vi "pulse detector tester_host vi.vi"() -> ()   [LabVIEW 2021]
uses:
  FPGA/PDW interpoter params.ctl
  FPGA/reciver params.ctl
  <vilib>/FPGAPlugInAG/USRP 294xR; 295xR 200 MSps/niLvFpga_Open_USRP 294xR; 295xR 200 MSps.vi
  <vilib>/rvi/interface/common/dynamic/niFpgaDynamicAddResources.vi
  <vilib>/rvi/interface/common/niFpgaWaitOnOcc.vi
  <vilib>/Utility/error.llb/Error Cluster From Error Code.vi
  <vilib>/rvi/errors/niLvFpgaAdjustHostInterfaceError.vi
  <vilib>/FPGAPlugInAG/Dynamic/niLvFpga_Close_Dynamic.vi
  <vilib>/rvi/interface/nirviOpenFPGA/nirviOpenFPGA.xnode
  FPGA Bitfiles/reciever_USRP294xR;295xR2_pulsedetectormai_nRNCtQH+qRA.lvbitx
  <vilib>/rvi/interface/nirviMethod/nirviMethod.xnode
  <vilib>/rvi/interface/nirviReadWriteControl/nirviReadWriteControl.xnode
  <vilib>/rvi/interface/nirviCloseFPGA/nirviCloseFPGA.xnode
  <vilib>/rvi/errors/niLvFpgaMergeErrorWithErrorCode.vi
  <vilib>/FPGAPlugInAG/Dynamic/niLvFpga_ReadFifo_Dynamic.vi
  NiFpgaLv.dll
  <vilib>/rvi/interface/Simulation/niFpgaSimulationCallBeginRW.vi
  <vilib>/FPGAPlugInAG/Dynamic/niLvFpga_WriteFifo_Dynamic.vi
  <vilib>/FPGAPlugInAG/Dynamic/niLvFpga_ConfigureFifo_Dynamic.vi
panel:
  out "num of pulses detected":i32
  in  "Tab Control 2":T1(tab)
  in  "F base (Hz)":u32 format="%.0p"
  in  "Fs  (Hz)":u32=80000000 format="%.0p"
  in  "Rx max gap (fft cycels)":u8
  in  "Rx max PW (fft cycels)":u16=30000
  in  "Rx min PW (fft cycels)":u16=6
  in  "Rx detection bar (dB)":dbl=120.0
  in  "where the  pulse detector run?":bool caption="run on fpga"
  in  "TDMS IQ file":path=path "C:/Users/NI/Desktop/RDC_chaim.tdms channel0.tdms"
  in  "lo likege removal (bins aruond 0)":i32=-1
  in  "max PW (fft cycels)":dbl=9999.0
  in  "min PW (fft cycels)":u16
  in  "min amp (dB)":dbl format="%_3p"
  out "frequncy resolotion (Hz)":dbl format="%#_3p"
  out "PW_resolotion (sec)":dbl format="%#_6p"
  out "spectrogram":sgl[][](graph)
  in  "Map selector":T2(ring)=enum."inverse grey"
  out "end of file?":bool
  in  "Next Button":bool
  out "PW":cluster{dbl[], dbl[]}(graph)
  out "amp(dB)/ frequncy (Hz)":cluster{dbl[], dbl[]}(graph)
  out "F (Hz)":cluster{dbl[], dbl[]}(graph)
  out "amp(dB)":cluster{dbl[], dbl[]}(graph)
  out "PDWs":T3(array[cluster]) {"t end (sec)" format="%#_6p"; "f(Hz)" format="%#_3p"; "PW (sec)" format="%#_6p"; "magnitude(dB)" format="%#_3g"}
  out "read parts":i32
  in  "off":bool
  out "streaming":bool
  # "Pulse Detector Tester"
  # "resolotions"
  # "This is \"pulse detector\" tester, the user shuold select a TDMS file\nwith some pulses on it and the VI will run it on FPGA or host in \norder to detect the pulses.\nthe reciver params are the parameters needed for the pulse detector:\n max gap - the maxiemom of undetected parts in the spot that \nthe detector keep loking for continuety.\nRx max PW - if the pulse is CW then we like to get  a PDW even if the pulse isnt done.\nRx min PW - less then this size is probbly just termal noise\nRx detection bar - the detection bar.\ndisplay filters could help the user make the presenting graphs easyer to understend."
  # "secnario params"
  # "reciever params"
  # "display filters"
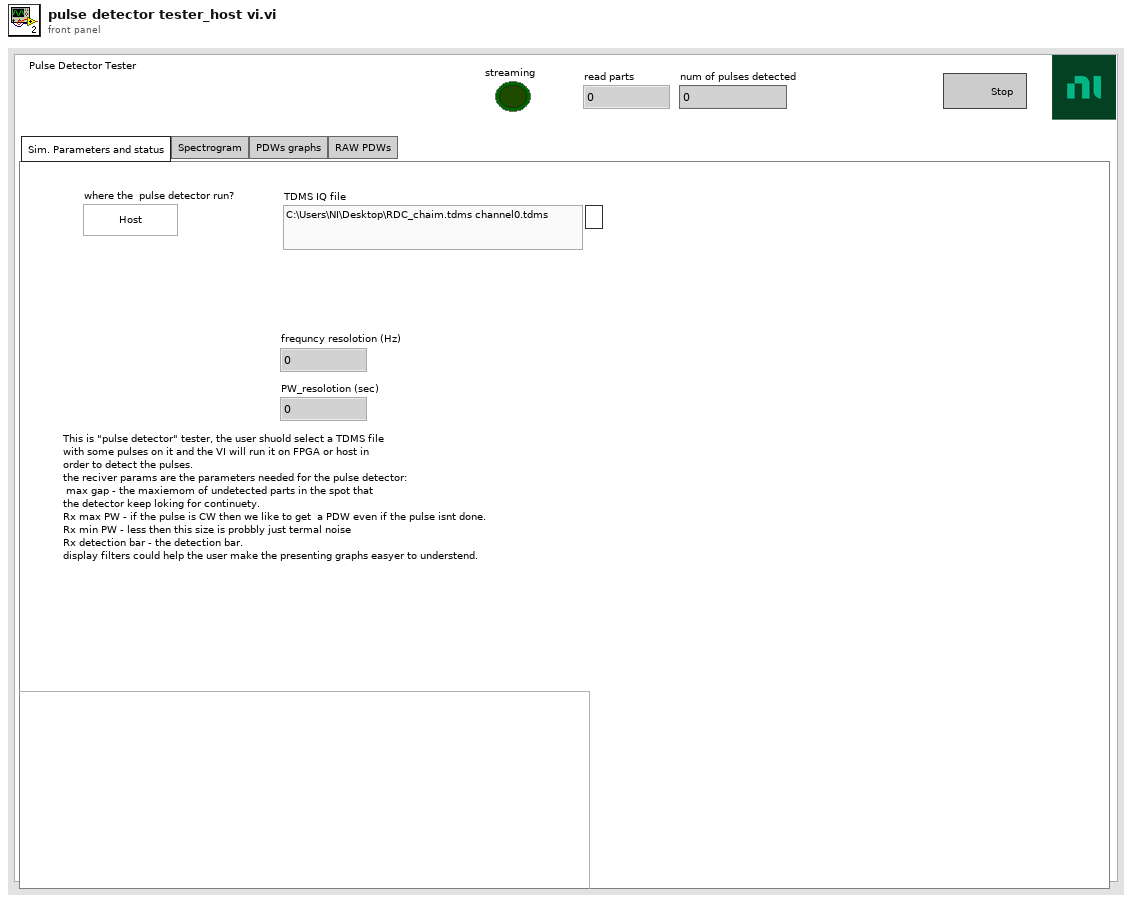
[diagram p1: front panel]
types:
  T1 = enum32{"Sim. Parameters and status", "Spectrogram", "PDWs graphs", "RAW PDWs"}
  T2 = enum16{"fire", "rainbow", "grey", "inverse grey", "ice", "original"}
  T3 = cluster{"f(Hz)":dbl, "PW (sec)":dbl, "magnitude(dB)":dbl, "t end (sec)":dbl}[]
  T4 = enum16{"open", "open or create", "create or replace", "create", "open (read-only)"}
  T5 = typedef "reciver params.ctl" = cluster{"min PW (fft cycels)":u16, "max PW (fft cycels)":u16, "max gap (fft cycels)":u8, "detection bar (liniar amp)":fxp<+,64,63>}
  T6 = typedef "PDW interpoter params.ctl" = cluster{"Fs (Hz)":u32, "fft size ":u32, "F base (Hz)":u32, "min AMP (dB)":dbl, "PW low bar (fft cycle)":dbl, "Pw high bar (fft cycle)":dbl, "lo likege removal (fft bin)":i32, "max gap (fft cycle)":dbl}
  T7 = typedef "specrogram_and_param.ctl" = cluster{"Array out":sgl[][], "start_ time":dbl, "min_amp":dbl, "amp_scale":dbl, "end of file":bool}
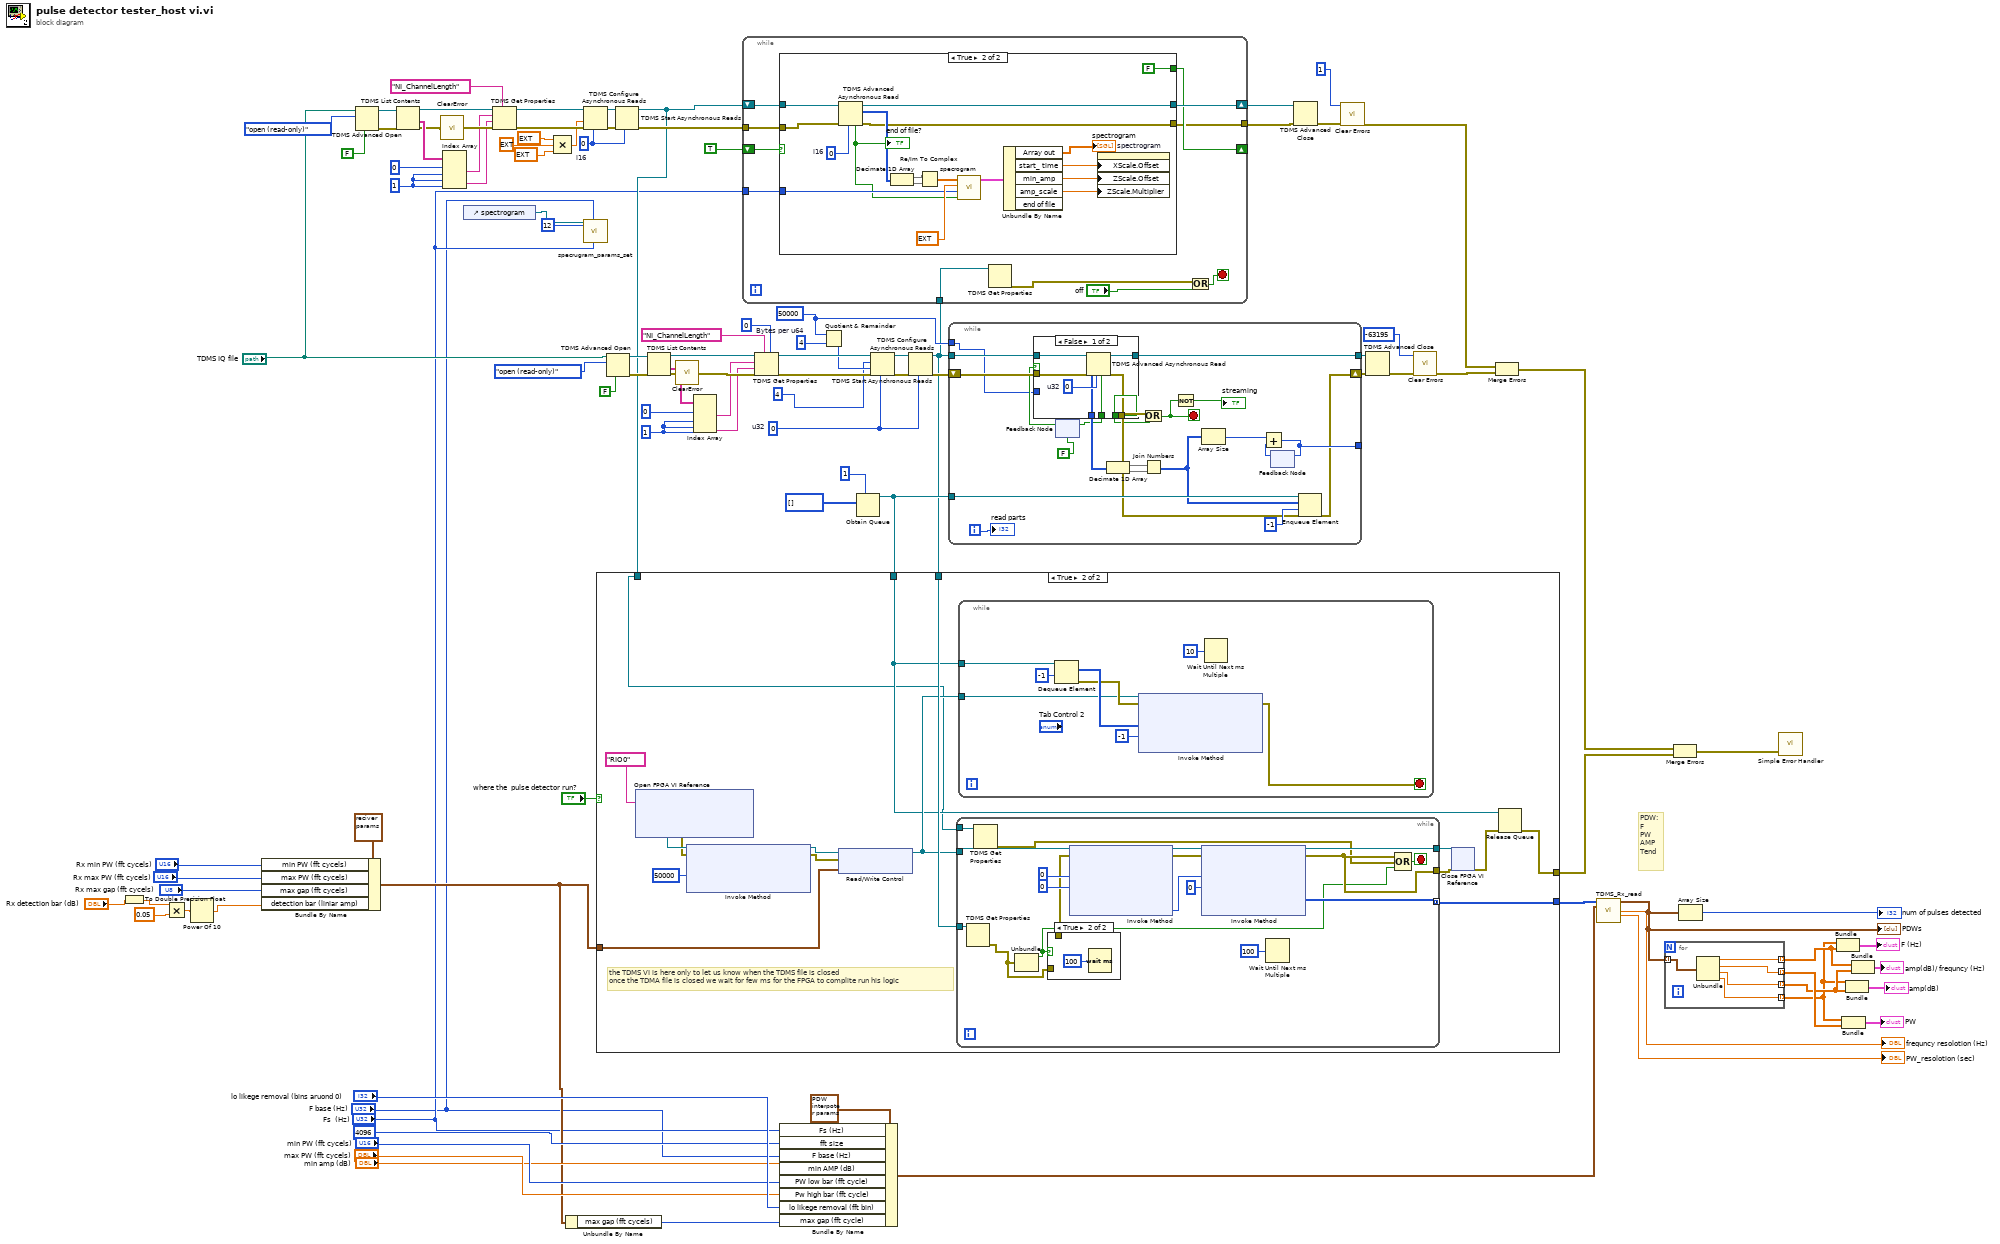
[diagram p0: block diagram]
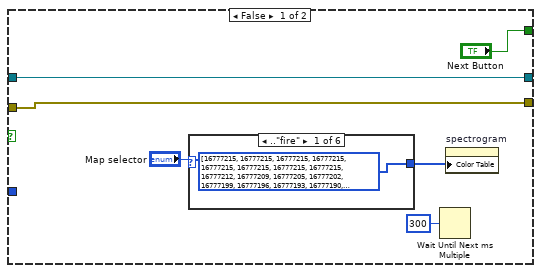
[diagram p2: hidden frame]
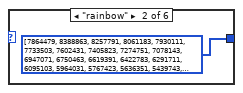
[diagram p3: hidden frame]
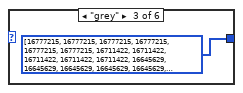
[diagram p4: hidden frame]
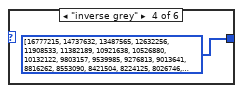
[diagram p5: hidden frame]
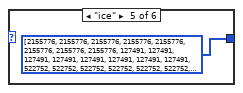
[diagram p6: hidden frame]
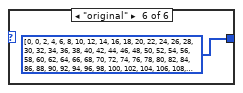
[diagram p7: hidden frame]
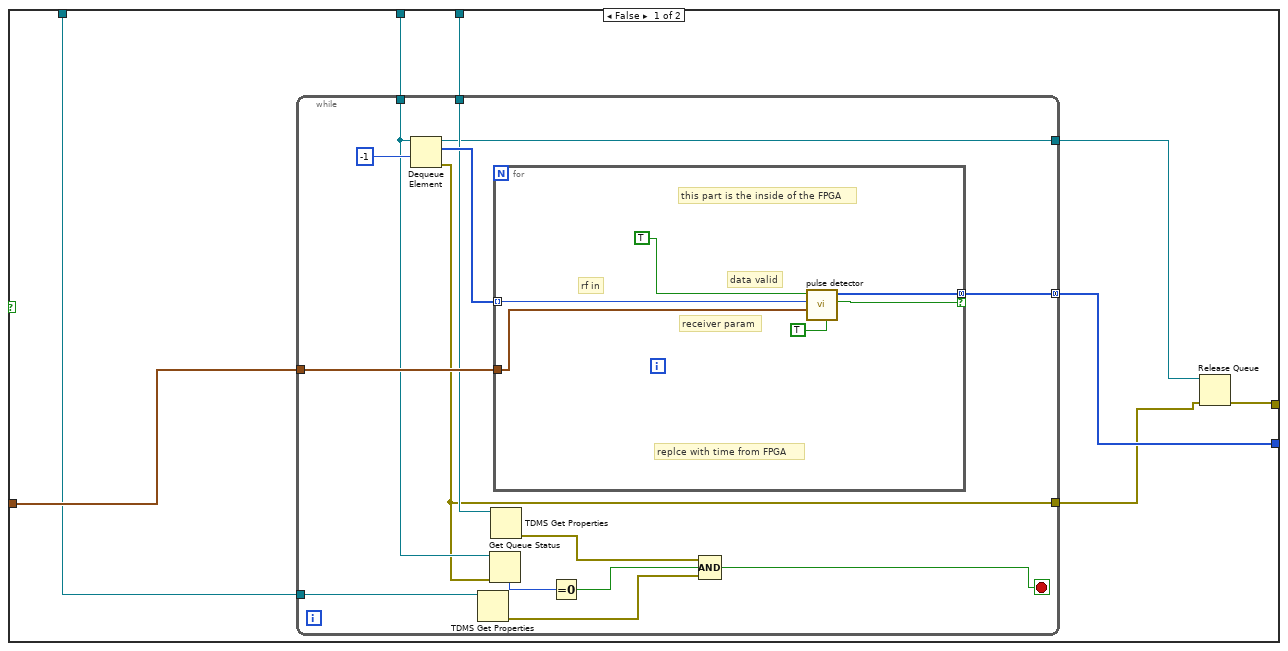
[diagram p8: hidden frame]
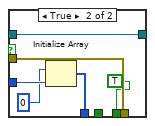
[diagram p10: hidden frame]
diagram:
  w24 = i16 0  # i16
  w40 = 1 ("disabled index (col)")
  w44 = u64 50000 ("Read Block Size (bytes)")
  w95 = 1 ("disabled index (col)")
  w83 = u64 4  # Bytes per u64
  w80 = i16 0  # u32
  # "PDW:\nF\nPW\nAMP\nTend"
  n1 = To Double Precision Float(number="Rx detection bar (dB)") -> (double precision float=w51:dbl)
  n2 = Multiply(x=w51, y=0.05) -> (x*y=w50:dbl)
  n3 = Power Of 10(x=w50) -> (10^x=w52:dbl)
  n4 = Bundle By Name(cluster=T5 {"min PW (fft cycels)"=5, "max PW (fft cycels)"=500, "max gap (fft cycels)"=1, "detection bar (liniar amp)"=1000000.0} ("reciver_params"), "min PW (fft cycels)"="Rx min PW (fft cycels)", "max PW (fft cycels)"="Rx max PW (fft cycels)", "max gap (fft cycels)"="Rx max gap (fft cycels)", "detection bar (liniar amp)"=w52) -> (w53:T5)
  n5 = TDMS Advanced Open(6:FALSE ("disable buffering? (T)"), 10:T4."open (read-only)" ("Operation"), 11:"TDMS IQ file") -> (0:w35:errorcluster, 3:w34:refnum<k34>)  [unwired: 2 in, 1 out]
  n6 = TDMS List Contents(4:w35, 7:w34) -> (0:w33:errorcluster, 1:w42:string[][], 3:w38:refnum<k34>)  [unwired: 1 in, 1 out]
  n7 = call <vilib>:"ClearError.vi"("error in (no error)"=w33) -> ("error out"=w39:errorcluster)
  n8 = Index Array(array=w42, index (row) #1=0 ("index (row)"), index (col) #1=w40, index (row) #2=w40, index (col) #2=w40) -> (element #1=w37:string, element #2=w31:string)
  n9 = control-ref of="spectrogram"() -> (w1:refnum<vi>)
  n10 = TDMS Get Properties(7:"NI_ChannelLength" ("property name"), 8:w39, 9:w31, 10:w37, 11:w38) -> (0:w30:errorcluster, 3:w29:refnum<k34>)  [unwired: 1 in, 4 out]
  n11 = Compound Arithmetic op=MULTIPLY(ext 4096.0 ("x"), ext 2.0 ("y"), ext 1500.0 ("value")) -> (w21:ext)
  n12 = Unbundle By Name(w53) -> ("max gap (fft cycels)"=w56:u8)
  n13 = TDMS Configure Asynchronous Reads(6:w24, 8:w30, 9:w21, 11:w29) -> (0:w22:errorcluster, 3:w23:refnum<k34>)  [unwired: 2 in]
  n14 = call "specrugram_params_set.vi"("fs"="Fs  (Hz)", "center frequncy"="F base (Hz)", "fft size in power of  in"=12, 11:w1) -> ()  [unwired: 3 in, 5 out]
  n15 = TDMS Advanced Open(6:FALSE ("disable buffering? (T)"), 10:T4."open (read-only)" ("Operation"), 11:"TDMS IQ file") -> (0:w88:errorcluster, 3:w87:refnum<k34>)  [unwired: 2 in, 1 out]
  n16 = TDMS Start Asynchronous Reads(6:w24, 8:w22, 11:w23) -> (0:w19:errorcluster, 3:w6:refnum<k34>)  [unwired: 1 in]
  n17 = TDMS List Contents(4:w88, 7:w87) -> (0:w82:errorcluster, 1:w97:string[][], 3:w93:refnum<k34>)  [unwired: 1 in, 1 out]
  n18 = call <vilib>:"ClearError.vi"("error in (no error)"=w82) -> ("error out"=w94:errorcluster)
  n19 = Index Array(array=w97, index (row) #1=0 ("index (row)"), index (col) #1=w95, index (row) #2=w95, index (col) #2=w95) -> (element #1=w92:string, element #2=w91:string)
  n20 = TDMS Get Properties(5:u32 0, 7:"NI_ChannelLength" ("property name"), 8:w94, 9:w91, 10:w92, 11:w93) -> (0:w85:errorcluster, 3:w86:refnum<k34>)  [unwired: 4 out]
  n21 = Bundle By Name(cluster=T6 {"Fs (Hz)"=200000000, "fft size "=4096, "F base (Hz)"=2000000000, "min AMP (dB)"=0.0, "PW low bar (fft cycle)"=0.0, "Pw high bar (fft cycle)"=7000.0, "lo likege removal (fft bin)"=-1, "max gap (fft cycle)"=0.0} ("PDW interpoter params"), "Fs (Hz)"="Fs  (Hz)", "fft size"=u32 4096, "F base (Hz)"="F base (Hz)", "min AMP (dB)"="min amp (dB)", "PW low bar (fft cycle)"="min PW (fft cycels)", "Pw high bar (fft cycle)"="max PW (fft cycels)", "lo likege removal (fft bin)"="lo likege removal (bins aruond 0)", "max gap (fft cycle)"=w56) -> (w62:T6)
  n22 = Quotient & Remainder(x=w44, y=w83) -> (floor(x/y)=w84:u64)  [unwired: 1 out]
  n23 = Obtain Queue(max queue size (-1, unlimited)=1, element data type=u32[] []) -> (queue out=w67:refnum<queue>)  [unwired: 3 in, 2 out]
  n24 = TDMS Configure Asynchronous Reads(6:w80, 8:w85, 9:w84, 10:u32 4 ("number of buffers (4)"), 11:w86) -> (0:w99:errorcluster, 3:w98:refnum<k34>)  [unwired: 1 in]
  n25 = TDMS Start Asynchronous Reads(6:w80, 8:w99, 11:w98) -> (0:w103:errorcluster, 3:w5:refnum<k34>)  [unwired: 1 in]
  n26 = case shown="True" "where the  pulse detector run?" {
    tunnel: w53 -> [w111 w147]
    tunnel: w5 -> [w108 w145]
    tunnel: [w107 w139] -> w65
    tunnel: [w110 w142] -> w68
    tunnel: w67 -> [w109 w138]
    tunnel: w6 -> [w104 w132]
    frame False {
      n27 = while {
        tunnel: w111 -> [w125]
        tunnel: [w124] -> w110 mode=concatenating
        tunnel: w109 -> [w121]
        tunnel: w108 -> [w117]
        tunnel: [w115] -> w106
        tunnel: [w114] -> w105
        tunnel: w104 -> [w113]
        stop <- w116 stop-if-true
        n28 = Dequeue Element(queue=w121, timeout in ms (-1)=-1) -> (queue out=w114:refnum<queue>, element=w122:u32[], error out=w115:errorcluster)  [unwired: 1 in, 1 out]
        n29 = TDMS Get Properties(11:w113) -> (0:w112:errorcluster)  [unwired: 5 in, 5 out]
        n30 = Get Queue Status(queue=w121, error in (no error)=w115) -> (# elements in queue=w120:i32)  [unwired: 1 in, 7 out]
        n31 = TDMS Get Properties(11:w117) -> (0:w118:errorcluster)  [unwired: 5 in, 5 out]
        n32 = for {
          tunnel: [w128] -> w124 mode=concatenating if=w129
          tunnel: w125 -> [w130]
          tunnel: w122 -> [w127] mode=indexing
          # "rf in"
          # "receiver param"
          # "data valid"
          # "replce with time from FPGA"
          # "this part is the inside of the FPGA"
          n33 = call "pulse detector.vi"("calculate timeing inside"=TRUE ("set timing inside"), "reciver_params"=w130, "IQ sampels"=w127, "input valid"=TRUE) -> ("output valid"=w129:bool, "data out"=w128:u64[])  [unwired: 6 in]
        }
        n34 = Equal To 0?(x=w120) -> (x = 0?=w119:bool)
        n35 = Compound Arithmetic op=AND(w118, w119, w112) -> (w116:bool)
      }
      n36 = Release Queue(queue=w105, error in (no error)=w106) -> (error out=w107:errorcluster)  [unwired: 1 in, 2 out]
    }
    frame True {
      # "the TDMS VI is here only to let us know when the TDMS file is closed\nonce the TDMA file is closed we wait for few ms for the FPGA to complite run his logic"
      n37 = xnode "Open FPGA VI Reference"("resource name"=tag "RIO0") -> ("FPGA VI Reference Out"=w137:refnum<k20>, "error out"=w136:errorcluster)  [unwired: 1 in]
      n38 = xnode "Invoke Method"("FPGA VI Reference In"=w137, "error in"=w136, "Requested Depth"=u32 50000) -> ("FPGA VI Reference Out"=w135:refnum<k20>, "error out"=w134:errorcluster)  [unwired: 1 out]
      n39 = xnode "Read/Write Control"("FPGA VI Reference In"=w135, "error in"=w134, "reciver_params"=w147) -> ("FPGA VI Reference Out"=w141:refnum<k20>)  [unwired: 1 out]
      n40 = while {
        tunnel: w141 -> [w171]
        tunnel: [w164] -> w143
        tunnel: [w163] -> w142 mode=concatenating
        tunnel: w145 -> [w159]
        tunnel: [w158] -> w144
        tunnel: w132 -> [w157]
        stop <- w165 stop-if-true
        n41 = TDMS Get Properties(11:w159) -> (0:w160:errorcluster)  [unwired: 5 in, 5 out]
        n42 = TDMS Get Properties(11:w157) -> (0:w156:errorcluster)  [unwired: 5 in, 5 out]
        n43 = Unbundle(w160) -> ("status"=w161:bool)  [unwired: 2 out]
        n44 = case shown="True" w161 {
          tunnel: [w174 _] -> w162
          tunnel: w160 -> [w174 _]
          frame False {
          }
          frame True {
            n45 = Wait (ms)(milliseconds to wait=u32 100) -> ()  [unwired: 1 out]
          }
        }
        n46 = xnode "Invoke Method"("FPGA VI Reference In"=w171, "error in"=w162, "Number of Elements"=u32 0, "Timeout (ms)"=0) -> ("FPGA VI Reference Out"=w170:refnum<k20>, "error out"=w166:errorcluster, "Elements Remaining"=w169:u32)  [unwired: 1 out]
        n47 = xnode "Invoke Method"("FPGA VI Reference In"=w170, "error in"=w166, "Number of Elements"=w169, "Timeout (ms)"=0) -> ("FPGA VI Reference Out"=w158:refnum<k20>, "error out"=w164:errorcluster, "Data"=w163:u64[])  [unwired: 1 out]
        n48 = Wait Until Next ms Multiple(millisecond multiple=u32 100) -> ()  [unwired: 1 out]
        n49 = Compound Arithmetic op=OR(w164, w156, w161) -> (w165:bool)
      }
      n50 = while {
        tunnel: w138 -> [w154]
        tunnel: w141 -> [w151]
        stop <- w150 stop-if-true
        n51 = Dequeue Element(queue=w154, timeout in ms (-1)=-1) -> (element=w153:u32[], error out=w152:errorcluster)  [unwired: 1 in, 2 out]
        n52 = xnode "Invoke Method"("FPGA VI Reference In"=w151, "error in"=w152, "Data"=w153, "Timeout (ms)"=-1) -> ("error out"=w150:errorcluster)  [unwired: 2 out]
        n53 = Wait Until Next ms Multiple(millisecond multiple=u32 10) -> ()  [unwired: 1 out]
      }
      n54 = xnode "Close FPGA VI Reference"("FPGA VI Reference In"=w144, "error in"=w143) -> ("error out"=w140:errorcluster)
      n55 = Release Queue(queue=w138, error in (no error)=w140) -> (error out=w139:errorcluster)  [unwired: 1 in, 2 out]
    }
  }
  n56 = while {
    tunnel: w19 -> [w184]
    tunnel: "Fs  (Hz)" -> [w183]
    shift-right: [w185] -> w28
    shift-left: w6 -> [w186]
    shift-right: [w181] -> _
    shift-left: TRUE -> [w182]
    tunnel: [w179] -> w15
    tunnel: w5 -> [w177]
    stop <- w180 stop-if-true
    n57 = case shown="True" w182 {
      tunnel: w186 -> [w190 w216]
      tunnel: [w190 w215] -> w185
      tunnel: w184 -> [w188 w214]
      tunnel: w183 -> [_ w202]
      tunnel: ["Next Button" FALSE] -> w181
      tunnel: [w188 w199] -> w179
      frame False {
        n58 = case shown="..\"fire\"" "Map selector" {
          tunnel: [u32[] [16777215, 16777215, 16777215, 16777215, 16777215, 16777215, 16777215, 16777215, 16777212, 16777209, 16777205, 16777202, 16777199, 16777196, 16777193, 16777190, 16777186, 16777183, 16777180, 16777177, 16777174, 16777170, 16777167, 16777164, 16777161, 16777158, 16777154, 16777151, 16777148, 16777145, 16777142, 16777139, 16777135, 16777132, 16777129, 16777126, 16777123, 16777119, 16777116, 16777113, 16777110, 16777107, 16777103, 16777100, 16777097, 16777094, 16777091, 16777088, 16777084, 16777081, 16777078, 16777075, 16777072, 16777068, 16777065, 16777062, 16777059, 16777056, 16777052, 16777049, 16777046, 16777043, 16777040, 16777037, 16777033, 16777030, 16777027, 16777024, 16777021, 16777017, 16777014, 16777011, 16777008, 16777005, 16777001, 16776998, 16776995, 16776992, 16776989, 16776986, 16776982, 16776979, 16776976, 16776973, 16776970, 16776966, 16776963, 16776960, 16776192, 16775424, 16774400, 16773632, 16772864, 16772096, 16771328, 16770560, 16769536, 16768768, 16768000, 16767232, 16766464, 16765440, 16764672, 16763904, 16763136, 16762368, 16761344, 16760576, 16759808, 16759040, 16758272, 16757504, 16756480, 16755712, 16754944, 16754176, 16753408, 16752384, 16751616, 16750848, 16750080, 16749312, 16748288, 16747520, 16746752, 16745984, 16745216, 16744448, 16743424, 16742656, 16741888, 16741120, 16740352, 16739328, 16738560, 16737792, 16737024, 16736256, 16735232, 16734464, 16733696, 16732928, 16732160, 16731392, 16730368, 16729600, 16728832, 16728064, 16727296, 16726272, 16725504, 16724736, 16723968, 16723200, 16722176, 16721408, 16720640, 16719872, 16719104, 16718336, 16717312, 16716544, 16715776, 16715008, 16714240, 16713216, 16712448, 16711680, 16515072, 16318464, 16056320, 15859712, 15663104, 15466496, 15269888, 15073280, 14811136, 14614528, 14417920, 14221312, 14024704, 13762560, 13565952, 13369344, 13172736, 12976128, 12713984, 12517376, 12320768, 12124160, 11927552, 11730944, 11468800, 11272192, 11075584, 10878976, 10682368, 10420224, 10223616, 10027008, 9830400, 9633792, 9371648, 9175040, 8978432, 8781824, 8585216, 8388608, 8126464, 7929856, 7733248, 7536640, 7340032, 7077888, 6881280, 6684672, 6488064, 6291456, 6029312, 5832704, 5636096, 5439488, 5242880, 5046272, 4784128, 4587520, 4390912, 4194304, 3997696, 3735552, 3538944, 3342336, 3145728, 2949120, 2686976, 2490368, 2293760, 2097152, 1900544, 1703936, 1441792, 1245184, 1048576, 851968, 655360, 393216, 196608, 65793, 65793, 65793, 65793, 65793, 65793, 65793, 65793, 0] ("256 fire") u32[] [7864479, 8388863, 8257791, 8061183, 7930111, 7733503, 7602431, 7405823, 7274751, 7078143, 6947071, 6750463, 6619391, 6422783, 6291711, 6095103, 5964031, 5767423, 5636351, 5439743, 5308671, 5112063, 4980991, 4784383, 4653311, 4456703, 4325631, 4129023, 3932415, 3801343, 3604735, 3473663, 3277055, 3145983, 2949375, 2818303, 2621695, 2490623, 2294015, 2162943, 1966335, 1835263, 1638655, 1507583, 1310975, 1179903, 983295, 852223, 655615, 524543, 327935, 196863, 511, 1791, 3071, 4351, 5631, 6911, 8191, 9471, 10751, 12031, 13311, 14591, 15871, 17151, 18431, 19711, 20991, 22271, 23551, 24831, 26111, 27391, 28671, 29951, 31231, 32511, 33791, 35071, 36351, 37631, 38911, 40191, 41471, 42751, 44031, 45311, 46591, 47871, 49151, 50431, 51711, 52991, 54271, 55551, 56831, 58111, 59391, 60671, 61951, 63231, 64511, 65532, 65527, 65522, 65517, 65512, 65507, 65502, 65497, 65492, 65487, 65482, 65477, 65472, 65467, 65462, 65457, 65452, 65447, 65442, 65437, 65432, 65427, 65422, 65417, 65412, 65407, 65402, 65397, 65392, 65387, 65382, 65377, 65372, 65367, 65362, 65357, 65352, 65347, 65342, 65337, 65332, 65327, 65322, 65317, 65312, 65307, 65302, 65297, 65292, 65287, 65282, 261888, 589568, 917248, 1244928, 1572608, 1900288, 2227968, 2555648, 2883328, 3211008, 3538688, 3866368, 4194048, 4521728, 4849408, 5177088, 5504768, 5832448, 6160128, 6487808, 6815488, 7143168, 7470848, 7798528, 8126208, 8453888, 8781568, 9109248, 9436928, 9764608, 10092288, 10419968, 10747648, 11075328, 11403008, 11730688, 12058368, 12386048, 12713728, 13041408, 13369088, 13696768, 14024448, 14352128, 14679808, 15007488, 15335168, 15662848, 15990528, 16318208, 16645888, 16775936, 16774656, 16773376, 16772096, 16770816, 16769536, 16768256, 16766976, 16765696, 16764416, 16763136, 16761856, 16760576, 16759296, 16758016, 16756736, 16755456, 16754176, 16752896, 16751616, 16750336, 16749056, 16747776, 16746496, 16745216, 16743936, 16742656, 16741376, 16740096, 16738816, 16737536, 16736256, 16734976, 16733696, 16732416, 16731136, 16729856, 16728576, 16727296, 16726016, 16724736, 16723456, 16722176, 16720896, 16719616, 16718336, 16717056, 16715776, 16714496, 16713216, 16711680] ("rainbow") u32[] [16777215, 16777215, 16777215, 16777215, 16777215, 16777215, 16711422, 16711422, 16711422, 16711422, 16711422, 16645629, 16645629, 16645629, 16645629, 16645629, 16645629, 16579836, 16579836, 16579836, 16579836, 16579836, 16514043, 16514043, 16514043, 16514043, 16514043, 16448250, 16448250, 16448250, 16448250, 16448250, 16316664, 16382457, 16382457, 16382457, 16382457, 16316664, 16316664, 16316664, 16316664, 16250871, 16250871, 16250871, 16250871, 16250871, 16185078, 16185078, 16185078, 16185078, 16119285, 16119285, 16119285, 16119285, 16119285, 16053492, 16053492, 16053492, 16053492, 15987699, 15987699, 15987699, 15987699, 15921906, 15987699, 15921906, 15921906, 15856113, 15856113, 15856113, 15856113, 15856113, 15790320, 15790320, 15790320, 15724527, 15724527, 15724527, 15724527, 15658734, 15658734, 15658734, 15658734, 15592941, 15592941, 15592941, 15592941, 15527148, 15527148, 15527148, 15461355, 15461355, 15461355, 15461355, 15395562, 15395562, 15395562, 15395562, 15329769, 15329769, 15329769, 15263976, 15263976, 15263976, 15198183, 15198183, 15198183, 15198183, 15132390, 15132390, 15132390, 15066597, 15066597, 15066597, 15000804, 15000804, 15000804, 14935011, 14935011, 14935011, 14869218, 14869218, 14869218, 14803425, 14803425, 14803425, 14737632, 14737632, 14671839, 14671839, 14671839, 14606046, 14606046, 14606046, 14540253, 14540253, 14540253, 14474460, 14474460, 14408667, 14408667, 14408667, 14342874, 14342874, 14277081, 14277081, 14277081, 14211288, 14211288, 14145495, 14145495, 14079702, 14079702, 14013909, 14013909, 14013909, 13948116, 13948116, 13882323, 13882323, 13816530, 13816530, 13750737, 13750737, 13684944, 13684944, 13619151, 13619151, 13553358, 13553358, 13487565, 13487565, 13421772, 13421772, 13355979, 13290186, 13290186, 13224393, 13224393, 13158600, 13092807, 13092807, 13027014, 13027014, 12961221, 12895428, 12895428, 12829635, 12763842, 12763842, 12698049, 12632256, 12566463, 12566463, 12500670, 12434877, 12434877, 12369084, 12303291, 12237498, 12171705, 12171705, 12105912, 12040119, 11974326, 11908533, 11842740, 11776947, 11711154, 11645361, 11579568, 11513775, 11447982, 11382189, 11316396, 11250603, 11184810, 11119017, 10987431, 10921638, 10855845, 10790052, 10658466, 10592673, 10461087, 10395294, 10329501, 10197915, 10066329, 10000536, 9868950, 9737364, 9605778, 9474192, 9342606, 9211020, 9079434, 8882055, 8750469, 8553090, 8421504, 8224125, 7960953, 7763574, 7500402, 7237230, 6974058, 6645093, 6316128, 5855577, 5395026, 4868682, 4210752, 3289650, 2105376, 0] ("256 log up") u32[] [16777215, 14737632, 13487565, 12632256, 11908533, 11382189, 10921638, 10526880, 10132122, 9803157, 9539985, 9276813, 9013641, 8816262, 8553090, 8421504, 8224125, 8026746, 7895160, 7697781, 7566195, 7434609, 7303023, 7171437, 7039851, 6908265, 6776679, 6710886, 6579300, 6447714, 6381921, 6316128, 6184542, 6118749, 5987163, 5921370, 5855577, 5789784, 5658198, 5592405, 5526612, 5460819, 5395026, 5329233, 5263440, 5197647, 5131854, 5066061, 5000268, 4934475, 4868682, 4802889, 4737096, 4671303, 4605510, 4605510, 4539717, 4473924, 4408131, 4342338, 4342338, 4276545, 4210752, 4210752, 4144959, 4079166, 4013373, 4013373, 3947580, 3881787, 3881787, 3815994, 3750201, 3750201, 3684408, 3684408, 3618615, 3552822, 3552822, 3487029, 3487029, 3421236, 3421236, 3355443, 3289650, 3289650, 3223857, 3223857, 3158064, 3158064, 3092271, 3092271, 3026478, 3026478, 2960685, 2960685, 2894892, 2894892, 2829099, 2829099, 2763306, 2763306, 2763306, 2697513, 2697513, 2631720, 2631720, 2565927, 2565927, 2500134, 2500134, 2500134, 2434341, 2434341, 2368548, 2368548, 2368548, 2302755, 2302755, 2236962, 2236962, 2236962, 2171169, 2171169, 2171169, 2105376, 2105376, 2105376, 2039583, 2039583, 1973790, 1973790, 1973790, 1907997, 1907997, 1907997, 1842204, 1842204, 1842204, 1776411, 1776411, 1776411, 1710618, 1710618, 1710618, 1644825, 1644825, 1644825, 1579032, 1579032, 1579032, 1579032, 1513239, 1513239, 1513239, 1447446, 1447446, 1447446, 1381653, 1381653, 1381653, 1381653, 1315860, 1315860, 1315860, 1315860, 1250067, 1250067, 1250067, 1184274, 1184274, 1184274, 1184274, 1118481, 1118481, 1118481, 1118481, 1052688, 1052688, 1052688, 1052688, 986895, 986895, 986895, 921102, 921102, 921102, 921102, 921102, 855309, 855309, 855309, 855309, 789516, 789516, 789516, 789516, 723723, 723723, 723723, 723723, 657930, 657930, 657930, 657930, 657930, 592137, 592137, 592137, 592137, 526344, 526344, 526344, 526344, 526344, 460551, 460551, 460551, 460551, 460551, 394758, 394758, 394758, 394758, 328965, 328965, 328965, 328965, 328965, 263172, 263172, 263172, 263172, 263172, 197379, 197379, 197379, 197379, 197379, 131586, 131586, 131586, 131586, 131586, 131586, 65793, 65793, 65793, 65793, 65793, 0, 0, 0, 0, 0, 0] ("256 log down") u32[] [2155776, 2155776, 2155776, 2155776, 2155776, 2155776, 2155776, 2155776, 127491, 127491, 127491, 127491, 127491, 127491, 127491, 127491, 522752, 522752, 522752, 522752, 522752, 522752, 522752, 522752, 64018, 64018, 64018, 64018, 64018, 64018, 64018, 64018, 63778, 63778, 63778, 63778, 63778, 63778, 63778, 63778, 63790, 63790, 63790, 63790, 63790, 63790, 63790, 63790, 63797, 63797, 63797, 63797, 63797, 63797, 63797, 63797, 63807, 63807, 63807, 63807, 63807, 63807, 63807, 63807, 64068, 64068, 64068, 64068, 64068, 64068, 64068, 64068, 63828, 63828, 63828, 63828, 63828, 63828, 63828, 63828, 63833, 63833, 63833, 63833, 63833, 63833, 63833, 63833, 63836, 63836, 63836, 63836, 63836, 63836, 63836, 63836, 63836, 63836, 63836, 63836, 63836, 63836, 63836, 63836, 61790, 61790, 61790, 61790, 61790, 61790, 61790, 61790, 58464, 58464, 58464, 58464, 58464, 58464, 58464, 58464, 55387, 55387, 55387, 55387, 55387, 55387, 55387, 55387, 51286, 51286, 51286, 51286, 51286, 51286, 51286, 51286, 47440, 47440, 47440, 47440, 47440, 47440, 47440, 47440, 40284, 40284, 40284, 40284, 40284, 40284, 40284, 40284, 34154, 34154, 34154, 34154, 34154, 34154, 34154, 34154, 28540, 28540, 28540, 28540, 28540, 28540, 28540, 28540, 20113, 20113, 20113, 20113, 20113, 20113, 20113, 20113, 12193, 12193, 12193, 12193, 12193, 12193, 12193, 12193, 12714, 12714, 12714, 12714, 12714, 12714, 12714, 12714, 7351, 7351, 7351, 7351, 7351, 7351, 7351, 7351, 4800, 4800, 4800, 4800, 4800, 4800, 4800, 4800, 195, 195, 195, 195, 195, 195, 195, 195, 189, 189, 189, 189, 189, 189, 189, 189, 183, 183, 183, 183, 183, 183, 183, 183, 175, 175, 175, 175, 175, 175, 175, 175, 164, 164, 164, 164, 164, 164, 164, 164, 155, 155, 155, 155, 155, 155, 155, 155] ("32 ice") u32[] [0, 0, 2, 4, 6, 8, 10, 12, 14, 16, 18, 20, 22, 24, 26, 28, 30, 32, 34, 36, 38, 40, 42, 44, 46, 48, 50, 52, 54, 56, 58, 60, 62, 64, 66, 68, 70, 72, 74, 76, 78, 80, 82, 84, 86, 88, 90, 92, 94, 96, 98, 100, 102, 104, 106, 108, 110, 112, 114, 116, 118, 120, 122, 124, 126, 128, 130, 132, 134, 136, 138, 140, 142, 144, 146, 148, 150, 152, 154, 156, 158, 160, 162, 164, 166, 168, 170, 172, 174, 176, 178, 180, 182, 184, 186, 188, 190, 192, 194, 196, 198, 200, 202, 204, 206, 208, 210, 212, 214, 216, 218, 220, 222, 224, 226, 228, 230, 232, 234, 236, 238, 240, 242, 244, 246, 248, 250, 252, 255, 131839, 263423, 395007, 526591, 658175, 789759, 921343, 1052927, 1184511, 1316095, 1447679, 1579263, 1710847, 1842431, 1974015, 2105599, 2237183, 2368767, 2500351, 2631935, 2763519, 2895103, 3026687, 3158271, 3289855, 3421439, 3553023, 3684607, 3816191, 3947775, 4079359, 4210943, 4342527, 4474111, 4605695, 4737279, 4868863, 5000447, 5132031, 5263615, 5395199, 5526783, 5658367, 5789951, 5921535, 6053119, 6184703, 6316287, 6447871, 6579455, 6711039, 6842623, 6974207, 7105791, 7237375, 7368959, 7500543, 7632127, 7763711, 7895295, 8026879, 8158463, 8290047, 8421631, 8553215, 8684799, 8816383, 8947967, 9079551, 9211135, 9342719, 9474303, 9605887, 9737471, 9869055, 10000639, 10132223, 10263807, 10395391, 10526975, 10658559, 10790143, 10921727, 11053311, 11184895, 11316479, 11448063, 11579647, 11711231, 11842815, 11974399, 12105983, 12237567, 12369151, 12500735, 12632319, 12763903, 12895487, 13027071, 13158655, 13290239, 13421823, 13553407, 13684991, 13816575, 13948159, 14079743, 14211327, 14342911, 14474495, 14606079, 14737663, 14869247, 15000831, 15132415, 15263999, 15395583, 15527167, 15658751, 15790335, 15921919, 16053503, 16185087, 16316671, 16448255, 16579839, 16777215] ("original")] -> w187
          frame .."fire" {
          }
          frame "rainbow" {
          }
          frame "grey" {
          }
          frame "inverse grey" {
          }
          frame "ice" {
          }
          frame "original" {
          }
        }
        n59 = Wait Until Next ms Multiple(millisecond multiple=u32 300) -> ()  [unwired: 1 out]
        n60 = property on="spectrogram" class="IntGraph (strict)"("Color Table"=w187) -> ()  [unwired: 2 in, 2 out]
      }
      frame True {
        w208 = i16 0  # i16
        n61 = TDMS Advanced Asynchronous Read(6:w208, 8:w214, 11:w216) -> (0:w199:errorcluster, 2:w212:i16[], 3:w215:refnum<k34>, 4:w201:bool)
        "end of file?" <- w201
        n62 = Decimate 1D Array(w212) -> (w211:i16[], w210:i16[])
        n63 = Re/Im To Complex(1:w210, 2:w211) -> (0:w209:cdb[])
        n64 = call "specrogram.vi"("end of file"=w201, "Fs"=w202, "fft size"=ext 4096.0, "Array in"=w209) -> ("specrogram"=w203:T7)  [unwired: 7 in]
        n65 = Unbundle By Name(w203) -> ("Array out"=→"spectrogram":sgl[][], "start_ time"=w204:dbl, "min_amp"=w207:dbl, "amp_scale"=w206:dbl)  [unwired: 1 out]
        n66 = property on="spectrogram" class="IntGraph (strict)"("XScale.Offset"=w204, "ZScale.Offset"=w207, "ZScale.Multiplier"=w206) -> ()  [unwired: 2 in, 2 out]
      }
    }
    n67 = TDMS Get Properties(11:w177) -> (0:w176:errorcluster)  [unwired: 5 in, 5 out]
    n68 = Or(x=w176, y="off") -> (x .or. y?=w180:bool)
  }
  n69 = while {
    tunnel: [w237] -> w101
    shift-right: [w227] -> w102
    shift-left: w103 -> [w238]
    tunnel: w5 -> [w236]
    tunnel: [w233] -> _
    tunnel: w67 -> [w230]
    tunnel: w44 -> [w218]
    i -> [w226]
    stop <- w235 stop-if-true
    n70 = feedback #1(FALSE ("read process finished?")) -> (w220:bool)
    n71 = case shown="False" w220 {
      tunnel: w238 -> [w245 w250]
      tunnel: [w244 w251] -> w237
      tunnel: w236 -> [w242 w251]
      tunnel: [w241 w250] -> w228
      tunnel: [w240 w248] -> w223
      tunnel: [w239 _] -> w222
      tunnel: [_ TRUE ("read process finished?")] -> w219
      tunnel: w218 -> [_ w247]
      frame False {
        w243 = i16 0  # u32
        n72 = TDMS Advanced Asynchronous Read(6:w243, 8:w245, 11:w242) -> (0:w241:errorcluster, 2:w240:i16[], 3:w244:refnum<k34>, 4:w239:bool)
      }
      frame True {
        n73 = Initialize Array(i16 0 ("Read Block Size (bytes)"), w247) -> (w248:i16[])
      }
    }
    n74 = feedback-in #1(w222) -> ()
    n75 = Decimate 1D Array(w223) -> (w225:i16[], w224:i16[])
    n76 = Or(x=w228, y=w219) -> (x .or. y?=w235:bool)
    n77 = Join Numbers(hi=w225, lo=w224) -> ((hi.lo)=w217:u32[])
    n78 = Not(x=w235) -> (.not. x?=→"streaming":bool)
    n79 = Array Size(array=w217) -> (size(s)=w232:i32)
    n80 = feedback #2() -> (w231:i32)  [unwired: 1 in]
    n81 = Add(x=w232, y=w231) -> (x+y=w233:i32)
    n82 = feedback-in #2(w233) -> ()
    n83 = Enqueue Element(queue=w230, element=w217, timeout in ms (-1)=-1, error in (no error)=w228) -> (error out=w227:errorcluster)  [unwired: 2 out]
    "read parts" <- w226
  }
  n84 = TDMS Advanced Close(8:w15, 11:w28) -> (0:w27:errorcluster)  [unwired: 2 in, 1 out]
  n85 = call <vilib>:"Clear Errors.vi"("error in (no error)"=w27, "specific error code to clear (0: all)"=1) -> ("error out"=w14:errorcluster)  [unwired: 4 in, 1 out]
  n86 = TDMS Advanced Close(8:w102, 11:w101) -> (0:w74:errorcluster)  [unwired: 2 in, 1 out]
  n87 = call <vilib>:"Clear Errors.vi"("error in (no error)"=w74, "specific error code to clear (0: all)"=-63195) -> ("error out"=w13:errorcluster)  [unwired: 4 in, 1 out]
  n88 = Merge Errors(w14, w13) -> (w12:errorcluster)
  n89 = call "TDMS_Rx_read.vi"("Array in"=w68, "PDW interpoter params"=w62) -> ("Array"=w11:cluster{dbl, dbl, "fixed-point":dbl, dbl}[], "frequncy resolotion"=→"frequncy resolotion (Hz)":dbl, "PW_resolotion"=→"PW_resolotion (sec)":dbl)  [unwired: 11 in]
  "PDWs" <- w11
  n90 = for {
    tunnel: w11 -> [w256] mode=indexing
    tunnel: [w255] -> w10 mode=indexing
    tunnel: [w254] -> w9 mode=indexing
    tunnel: [w253] -> w8 mode=indexing
    tunnel: [w252] -> w7 mode=indexing
    n91 = Unbundle(w256) -> (w255:dbl, w254:dbl, "fixed-point"=w253:dbl, w252:dbl)
  }
  n92 = Merge Errors(w12, w65) -> (w63:errorcluster)
  n93 = Array Size(array=w11) -> (size(s)=→"num of pulses detected":i32)
  n94 = call <vilib>:"Simple Error Handler.vi"("error in (no error)"=w63) -> ()  [unwired: 4 in, 5 out]
  n95 = Bundle(w7, w10) -> (→"F (Hz)":cluster{dbl[], dbl[]})  [unwired: 1 in]
  n96 = Bundle(w7, w9) -> (→"PW":cluster{dbl[], dbl[]})  [unwired: 1 in]
  n97 = Bundle(w7, w8) -> (→"amp(dB)":cluster{dbl[], dbl[]})  [unwired: 1 in]
  n98 = Bundle(w10, w8) -> (→"amp(dB)/ frequncy (Hz)":cluster{dbl[], dbl[]})  [unwired: 1 in]
